vi "Common TearDown.vi"(8 "error in (no error)":errorcluster, 11 "1553 Test in":refnum<class "1553 Test.lvclass">) -> (0 "error out":errorcluster, 3 "1553 Test out":refnum<class "1553 Test.lvclass">)   [LabVIEW 2016, in "1553 Test.lvclass"]
uses:
  1553 Test.lvclass
  Utilities/Simulated FPGA/FPGA Sim.lvclass
  1553 Test.lvclass/1553 Test.ctl
  1553 Board/1553 Board.lvclass
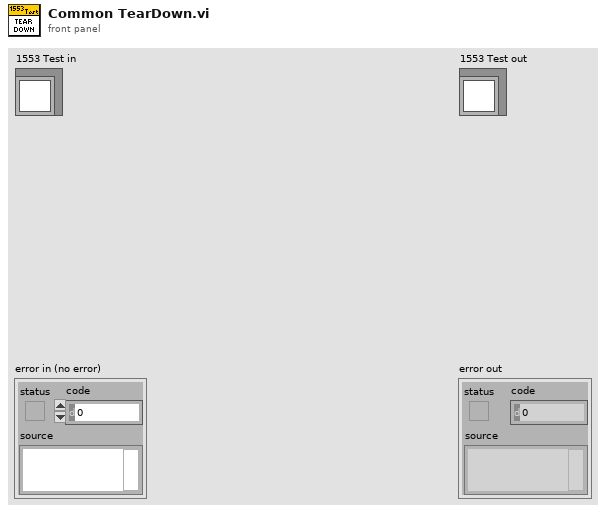
[diagram p1: front panel]
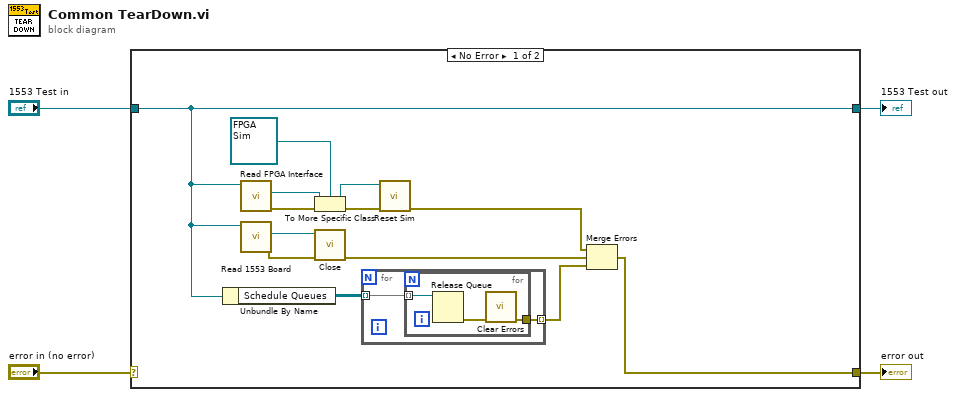
[diagram p0: block diagram]
diagram:
  n1 = case shown="No Error" "error in (no error)" {
    selector: "error in (no error)" -> [_ w24]
    tunnel: [w8 w24] -> w3
    tunnel: [w7 w23] -> w1
    tunnel: "1553 Test in" -> [w7 w23]
    frame No Error {
      n2 = Unbundle By Name(w7) -> ("Schedule Queues"=w6:refnum<queue>[][])
      n3 = call-dynamic "Read FPGA Interface.vi"("1553 Test in"=w7) -> ("error out"=w13:errorcluster, "FPGA Interface"=w17:refnum<class "FPGA Interface.lvclass">)  [unwired: 8 in, 1 out]
      n4 = call-dynamic "Read 1553 Board.vi"("1553 Test in"=w7) -> ("error out"=w14:errorcluster, "1553 Board"=w15:refnum<class "1553 Board.lvclass">)  [unwired: 8 in, 1 out]
      n5 = To More Specific Class(target class=refnum<class "FPGA Sim.lvclass"> refnum ("FPGA Sim.lvclass"), reference=w17, error in=w13) -> (specific class reference=w11:refnum<class "FPGA Sim.lvclass">, error out=w12:errorcluster)
      n6 = call-dynamic "Close.vi"("error in (no error)"=w14, "1553 Board in"=w15) -> ("error out"=w9:errorcluster)  [unwired: 9 in]
      n7 = for {
        tunnel: w6 -> [w18] mode=indexing
        tunnel: [w19] -> w5 mode=indexing
        n8 = for {
          tunnel: [w21] -> w19
          tunnel: w18 -> [w20] mode=indexing
          n9 = Release Queue(queue=w20) -> (error out=w22:errorcluster)  [unwired: 2 in, 2 out]
          n10 = call <vilib>:"Clear Errors.vi"("error in (no error)"=w22) -> ("error out"=w21:errorcluster)  [unwired: 5 in, 1 out]
        }
      }
      n11 = call-dynamic "Reset Sim.vi"("error in (no error)"=w12, "FPGA Sim in"=w11) -> ("error out"=w10:errorcluster)  [unwired: 8 in, 1 out]
      n12 = Merge Errors(w10, w9, w5) -> (w8:errorcluster)
    }
    frame Error {
    }
  }
  "error out" <- w3
  "1553 Test out" <- w1
